vi "Compra.vi"(8 "error in (no error)":errorcluster, 11 "Coffee Actor in":refnum<class "Coffee Actor.lvclass">) -> (0 "error out":errorcluster, 3 "Coffee Actor out":refnum<class "Coffee Actor.lvclass">)   [LabVIEW 2019, in "Coffee Actor.lvlib" / "Coffee Actor.lvclass"]
uses:
  Coffee Actor.lvclass
  C:/Program Files/National Instruments/LabVIEW 2019/vi.lib/ActorFramework/Actor/Actor.lvclass
  <vilib>/ActorFramework/Actor/Actor.lvclass/Actor.ctl
  Coffee Actor.lvclass/Coffee Actor.ctl
  UI Actor Messages/Compra Msg/Compra Msg.lvclass/Compra Msg.ctl
  <vilib>/ActorFramework/Message Enqueuer/Message Enqueuer.lvclass/Message Enqueuer.ctl
  <vilib>/ActorFramework/Message Enqueuer/Enqueue.vi
  UI Actor Messages/Compra Msg/Compra Msg.lvclass
  C:/Program Files/National Instruments/LabVIEW 2019/vi.lib/ActorFramework/Message/Message.lvclass
  <vilib>/ActorFramework/Message Priority Queue/Priority Enqueue.vi
  <vilib>/ActorFramework/Actor/Actor.lvclass
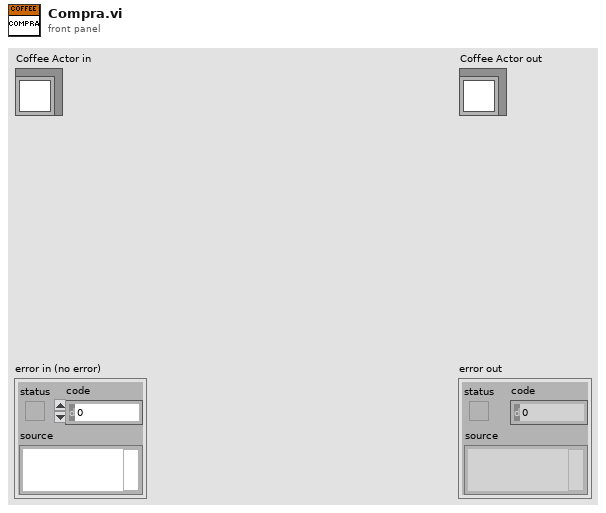
[diagram p1: front panel]
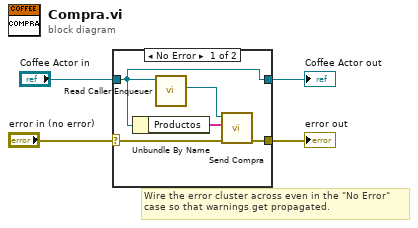
[diagram p0: block diagram]
diagram:
  # "Wire the error cluster across even in the \"No Error\"\ncase so that warnings get propagated."
  n1 = case shown="No Error" "error in (no error)" {
    selector: "error in (no error)" -> [w6 w11]
    tunnel: [w5 w11] -> w3
    tunnel: [w8 w10] -> w1
    tunnel: "Coffee Actor in" -> [w8 w10]
    frame No Error {
      n2 = Unbundle By Name(w8) -> ("Productos"=w9:string[])
      n3 = call <vilib>:"Read Caller Enqueuer.vi"("Actor"=w8) -> ("Caller Enqueuer"=w7:refnum<class "Message Enqueuer.lvclass">)  [unwired: 10 in]
      n4 = call "Send Compra.vi"("error in (no error)"=w6, "Producto"=w9, "Message Enqueuer"=w7) -> ("error out"=w5:errorcluster)  [unwired: 7 in, 1 out]
    }
    frame Error {
    }
  }
  "error out" <- w3
  "Coffee Actor out" <- w1
